vi "Pulse Generator 3.vi"(0 "Total Time":dbl=1500.0, 1 "EPR file path":path=path "C:/Users/Ouyang Group/Documents/Data/8-10-15/test", 3 "Z Pos":dbl=51.3, 4 "Pule Sequence file path":path=path "C:/Users/Ouyang Group/Documents/Data/8-6-15/T1 pulse sequence", 5 "X Pos":dbl=98.0, 7 "Y pos":dbl=76.0, 8 "start/restart":bool, 9 "track and epr":bool, 11 "Z-track?":bool, 12 "load":bool, 13 "Y Parameters":T1={"Number of Y Steps"=200, "Max Y (V)"=2.0, "Min Y (V)"=-2.0}, 16 "Tracking Interval":dbl=150.0, 17 "Tab Control":T3(tab)=enum."T1", 19 "X Parameters":T2={"Number of X Steps"=200, "Max X (V)"=2.0, "Min X (V)"=-2.0}, 20 "Rest time Min":dbl=2e-08, 21 "Rest time Max":dbl=0.0002, 25 "Rest time No. Steps":i32=20, 27 "type":u16(ring)=1 items=["Linear", "Logarithmic"]) -> (15 "Y Position":dbl=8.403706365395546, 23 "Z Position":dbl=77.35, 24 "X Position":dbl=39.29989668925261)   [LabVIEW 2012]
uses:
  <vilib>/Utility/file.llb/Write To Spreadsheet File (DBL).vi
panel:
  in  "CW for Tracking?":bool
  in  "Stop Program":bool
  out "EPR":bool
  out "Tracking Loop":dbl=6.0
  out "Track":bool
  out "Cross Section Y":dbl[](graph)=[21.0, 21.0, 22.0, 23.0, 28.0, 18.0, 27.0, 23.0, 21.0, 23.0, 27.0, 24.0, 27.0, 48.0, 72.0, 155.0, 223.0, 269.0, 346.0, 310.0, 298.0, 201.0, 115.0, 77.0, 45.0, 31.0, 30.0, 22.0, 20.0, 22.0, 23.0, 32.0, 17.0, 24.0, 22.0, 22.0, 31.0, 30.0, 37.0]
  out "Cross Section X":dbl[](graph)=[40.0, 23.0, 29.0, 30.0, 20.0, 26.0, 17.0, 31.0, 49.0, 64.0, 98.0, 144.0, 182.0, 231.0, 269.0, 259.0, 260.0, 248.0, 193.0, 187.0, 133.0, 113.0, 84.0, 52.0, 39.0, 24.0, 24.0, 33.0, 19.0, 20.0, 16.0, 21.0, 26.0, 30.0, 25.0, 26.0, 20.0, 24.0, 24.0]
  out "Gave up?":bool
  in  "RS232 settings":cluster{"Portnumber":i32, "Baudrate":u16}={"Portnumber"=6, "Baudrate"=5} {"Portnumber" items=["COM1", "COM2", "COM3", "COM4", "COM5", "COM6", "COM7", "COM8", "COM9", "COM10", "COM11", "COM12", "COM13", "COM14", "COM15", "COM16", "COM17", "COM18", "COM19", "COM20", "COM21", "COM22", "COM23", "COM24", "COM25", "COM26", "COM27", "COM28", "COM29", "COM30"]; "Baudrate" items=["9600", "14400", "19200", "38400", "57600", "115200"]}
  in  "ref?":bool=TRUE
  in  "MW Delay":dbl=5e-08
  in  "Sig/Ref pause":dbl=5e-07
  in  "Rate (Hz)":dbl=2.0
  in  "Pulse MW":bool
  in  "Pulse Laser":bool
  in  "Delay Blocks":u16=4
  in  "Divide By":u16(ring) items=["1", "8", "16", "32"]
  in  "MW width Min":dbl=2e-08
  in  "MW width step size":dbl=5e-09
  in  "MW width Max":dbl=5e-07
  in  "Rabi Freq":dbl=7000000.0
  in  "Tau Max":dbl=0.001
  in  "Tau Min":dbl=2e-08
  in  "Tau No. Steps":i32=20
  in  "type 2":u16(ring)=1 items=["Linear", "Logarithmic"]
  in  "T1 APD width":dbl=5e-07
  in  "T1 Signal Delay":dbl=6e-07
  in  "T1 AOM length":dbl=2.5e-06
  in  "T1 AOM Rest":dbl=1e-06
  in  "Pi Pulse?":bool
  in  "Tau step size":dbl
  in  "Tau max":dbl
  in  "Tau min":dbl
  in  "Rabi Frequency":dbl
  in  "Pulse offset 2":dbl
  in  "Rabi Frequency":dbl
  in  "Tau max":dbl
  in  "Tau min":dbl
  in  "Tau step size":dbl
  in  "Equal Pulse length":bool
  in  "Pulse offset":dbl
  in  "Tau":dbl
  in  "Rabi Frequency  2":dbl
  in  "Tau' max 2":dbl
  in  "Tau' min 2":dbl
  in  "Tau' step size 2":dbl
  in  "Rabi Frequency":dbl
  in  "Tau min":dbl
  in  "Tau max":dbl
  in  "Tau step size":dbl
  in  "No. Pi Pulses":i32
  in  "Pulse offset":dbl
  in  "0->+?":bool
  in  "AOM Rest time":dbl=1e-06
  in  "Signal delay":dbl=7.2e-07
  in  "N Loop":i32=10000
  in  "APD signal width":dbl=3e-07
  out "Run":bool
  out "Scan size":i32
  in  "AOM Pulse length":dbl=2.5e-06
  in  "Path to spinapi.dll":path=path "C:/SpinCore/SpinAPI/dll/spinapi64.dll"
  in  "stop":bool
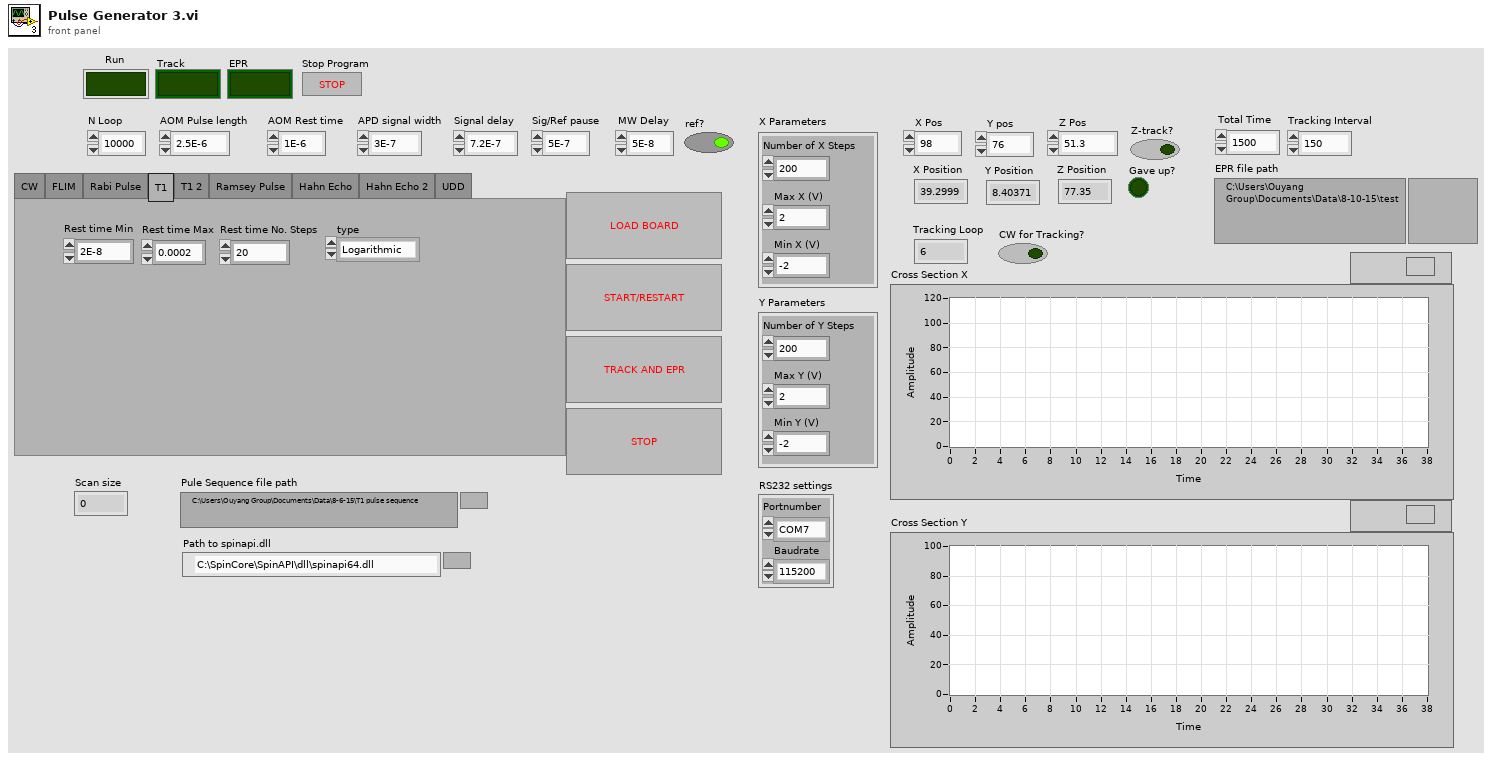
[diagram p1: front panel]
types:
  T1 = cluster{"Number of Y Steps":i32, "Max Y (V)":dbl, "Min Y (V)":dbl}
  T2 = cluster{"Number of X Steps":i32, "Max X (V)":dbl, "Min X (V)":dbl}
  T3 = enum32{"CW", "FLIM", "Rabi Pulse", "T1", "T1 2", "Ramsey Pulse", "Hahn Echo", "Hahn Echo 2", "UDD"}
  T4 = cluster{"Instruct Data":i32, "Op Code":i32, "Flags":bool[], "Comments":string, "Time (s)":dbl}
  T5 = enum16{"Pulse Program", "Frequency Registers", "TX Phase Registers", "RX Phase Registers"}
  T6 = cluster{"Instruct Data":i32, "Op Code":i32, "Flags":bool[], "Comments":string, "Time (s)":dbl}[]
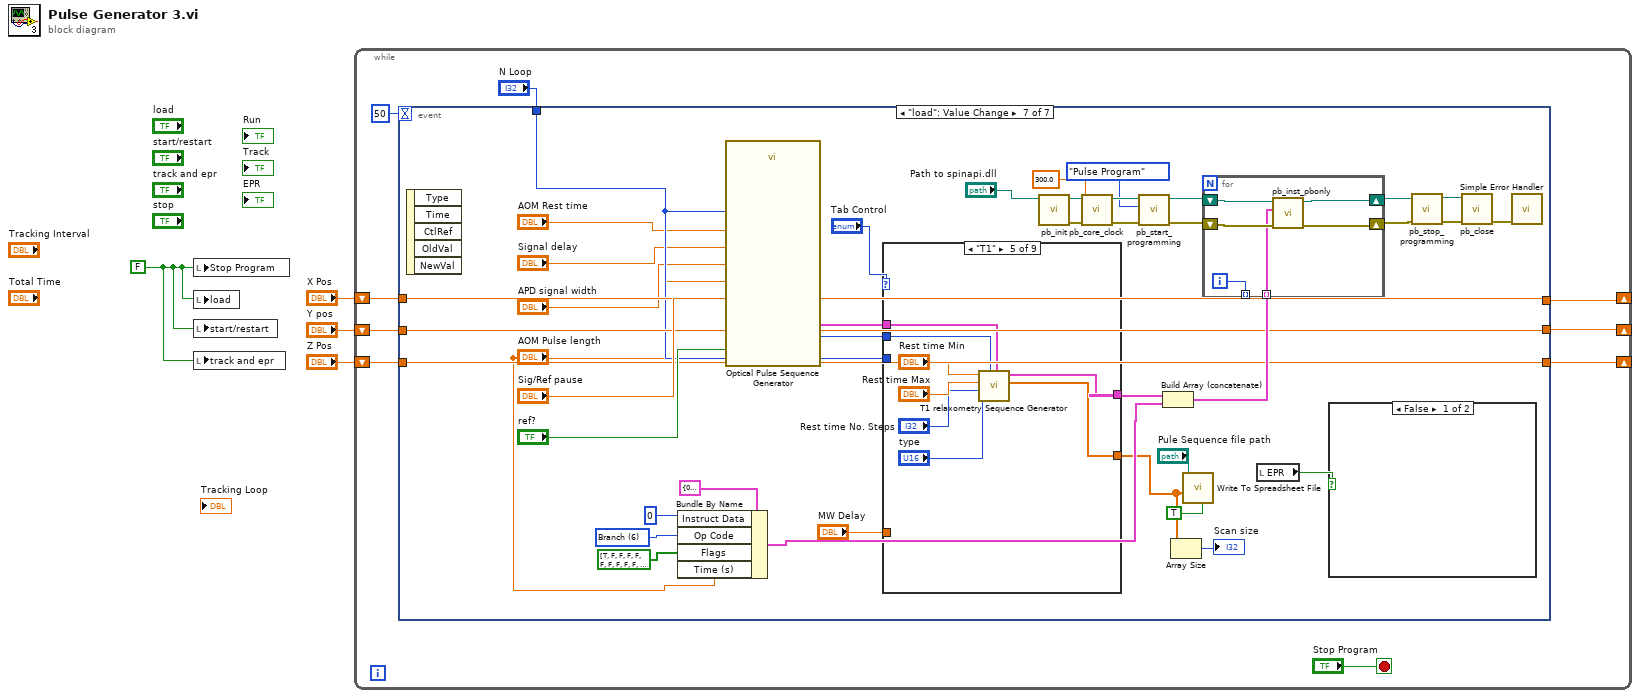
[diagram p0: block diagram]
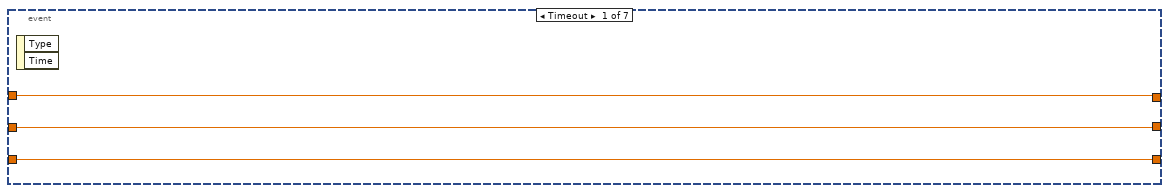
[diagram p2: hidden frame]
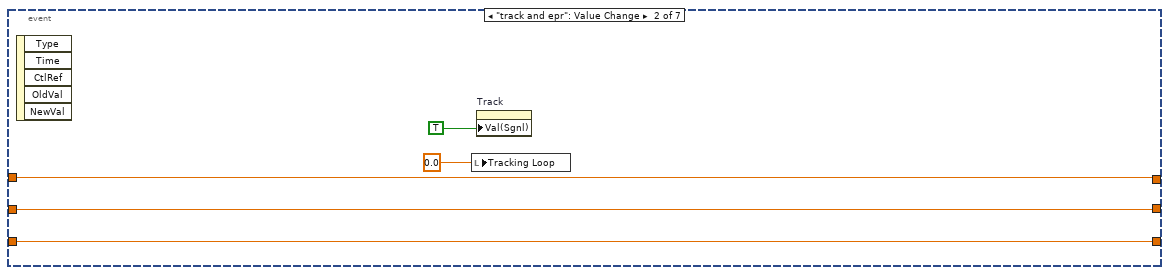
[diagram p3: hidden frame]
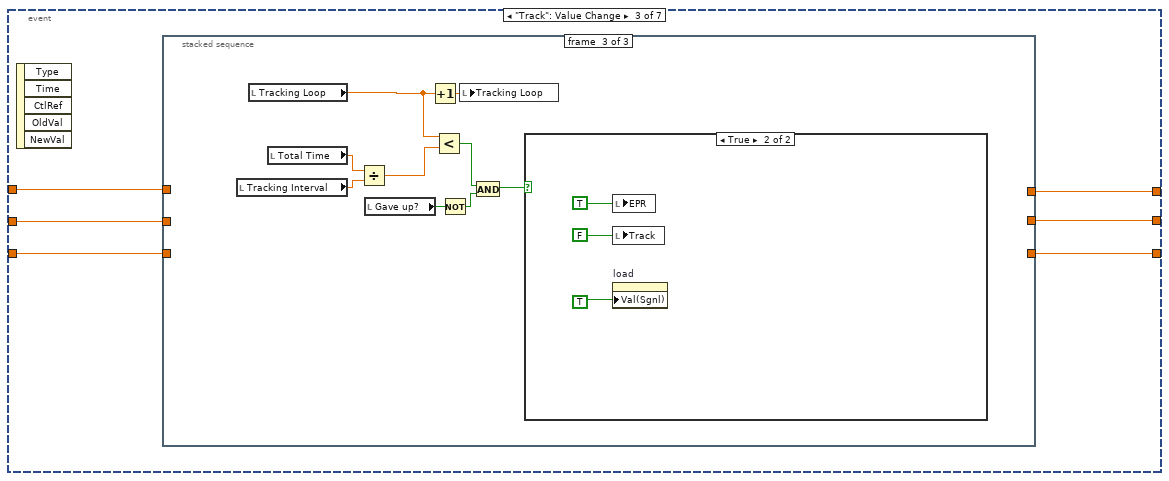
[diagram p4: hidden frame]
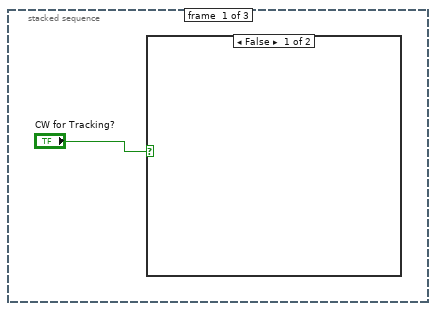
[diagram p5: hidden frame]
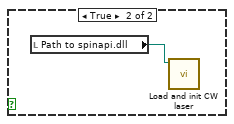
[diagram p6: hidden frame]
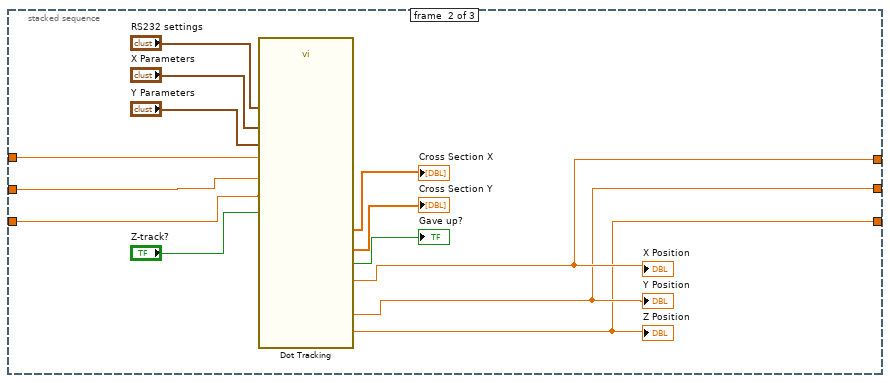
[diagram p7: hidden frame]
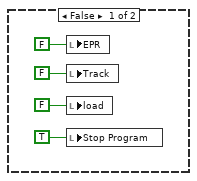
[diagram p8: hidden frame]
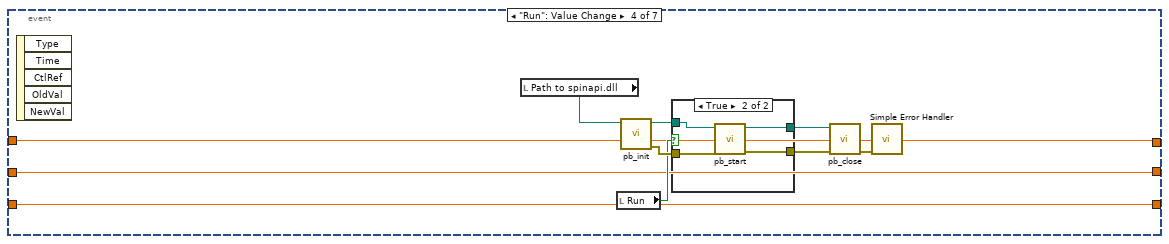
[diagram p9: hidden frame]
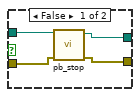
[diagram p10: hidden frame]
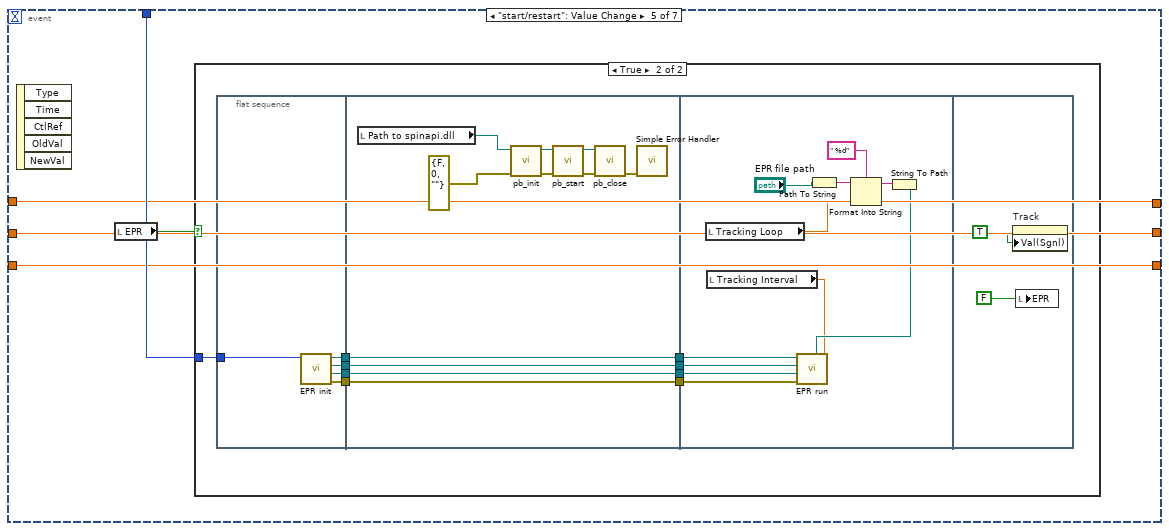
[diagram p11: hidden frame]
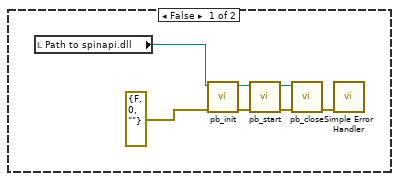
[diagram p12: hidden frame]
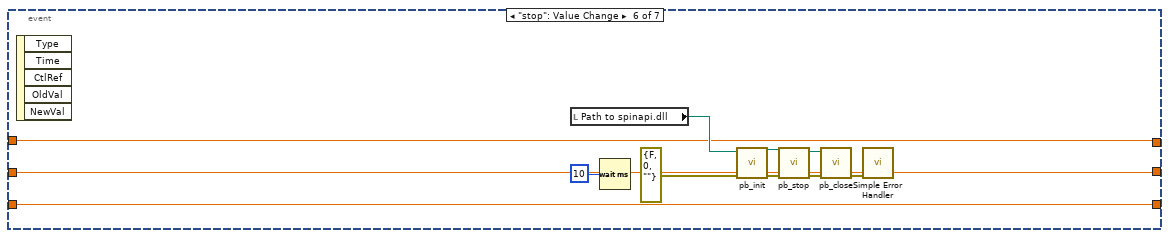
[diagram p13: hidden frame]
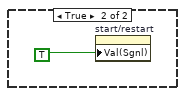
[diagram p14: hidden frame]
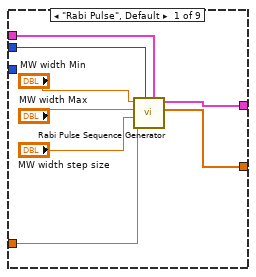
[diagram p15: hidden frame]
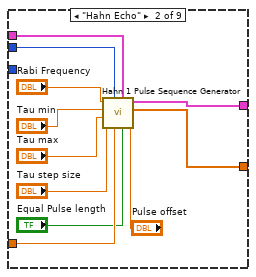
[diagram p16: hidden frame]
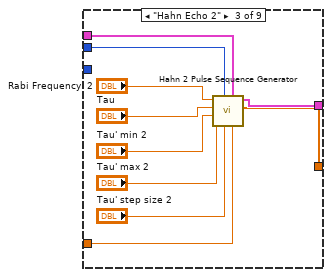
[diagram p17: hidden frame]
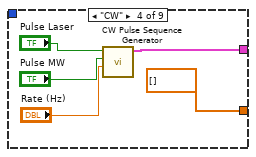
[diagram p18: hidden frame]
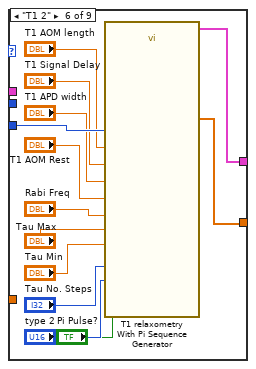
[diagram p19: hidden frame]
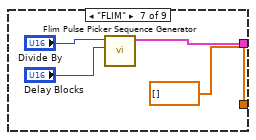
[diagram p20: hidden frame]
diagram:
  w4 = FALSE ("Stop Program")
  n1 = local write "Stop Program"(w4) -> ()
  n2 = local write "load"(w4) -> ()
  n3 = local write "start/restart"(w4) -> ()
  n4 = local write "track and epr"(w4) -> ()
  n5 = while {
    shift-right: [w7] -> _
    shift-left: "X Pos" -> [w10]
    shift-right: [w6] -> _
    shift-left: "Y pos" -> [w9]
    shift-right: [w5] -> _
    shift-left: "Z Pos" -> [w8]
    stop <- "Stop Program" stop-if-true
    n6 = event shown="[6] \"load\": Value Change" {
      selector: _ -> [_ _ _ _ _ _ _]
      dyn-events: _ -> [_ _ _ _ _ _ _]
      timeout: 50 -> [_ _ _ _ _ _ _]
      tunnel: "N Loop" -> [_ _ _ _ w80 _ w142]
      tunnel: w10 -> [w16 w19 w27 w61 w79 w129 w145]
      tunnel: w9 -> [w15 w18 w26 w60 w78 w128 w144]
      tunnel: w8 -> [w14 w17 w25 w59 w77 w127 w143]
      tunnel: [w16 w19 w24 w61 w79 w129 w145] -> w7
      tunnel: [w15 w18 w23 w60 w78 w128 w144] -> w6
      tunnel: [w14 w17 w22 w59 w77 w127 w143] -> w5
      event Timeout {
        n7 = event-data() -> ()  [unwired: 1 in, 2 out]
      }
      event "track and epr": Value Change {
        n8 = event-data() -> ()  [unwired: 1 in, 5 out]
        n9 = local write "Tracking Loop"(0.0 ("Tracking Loop")) -> ()
        n10 = property on="Track" class="Bool (strict)"("Val(Sgnl)"=TRUE ("Track")) -> ()  [unwired: 2 in, 2 out]
      }
      event "Track": Value Change {
        n11 = event-data() -> ()  [unwired: 1 in, 5 out]
        n12 = stacked-sequence {
          tunnel: w27 -> [_ w35 _]
          tunnel: w26 -> [_ w34 _]
          tunnel: w25 -> [_ w33 _]
          tunnel: [_ w32 _] -> w24
          tunnel: [_ w31 _] -> w23
          tunnel: [_ w30 _] -> w22
          frame #0 {
            n13 = case shown="False" "CW for Tracking?" {
              frame False {
              }
              frame True {
                n14 = local read "Path to spinapi.dll"() -> (w29:path)
                n15 = call "Load and init CW laser.vi"("path in"=w29) -> ()  [unwired: 11 in]
              }
            }
          }
          frame #1 {
            n16 = call "Dot Tracking.vi"("X"="X Parameters", "Y Parameters"="Y Parameters", "RS232 settings"="RS232 settings", "X Pos"=w35, "Y pos"=w34, "Z Pos"=w33, "Z-track?"="Z-track?") -> ("X Position"=w32:dbl, "Y Position"=w31:dbl, "Z Position"=w30:dbl, "Cross Section X"=→"Cross Section X":dbl[], "Cross Section Y"=→"Cross Section Y":dbl[], "Gave up?"=→"Gave up?":bool)  [unwired: 2 in, 1 out]
            "X Position" <- w32
            "Y Position" <- w31
            "Z Position" <- w30
          }
          frame #2 {
            n17 = local read "Tracking Interval"() -> (w51:dbl)
            n18 = local read "Tracking Loop"() -> (w44:dbl)
            n19 = local read "Total Time"() -> (w50:dbl)
            n20 = Divide(x=w50, y=w51) -> (x/y=w49:dbl)
            n21 = local read "Gave up?"() -> (w47:bool)
            n22 = Increment(x=w44) -> (x+1=w43:dbl)
            n23 = Less?(x=w44, y=w49) -> (x < y?=w48:bool)
            n24 = Not(x=w47) -> (.not. x?=w45:bool)
            n25 = local write "Tracking Loop"(w43) -> ()
            n26 = And(x=w48, y=w45) -> (x .and. y?=w46:bool)
            n27 = case shown="True" w46 {
              frame False {
                n28 = local write "EPR"(FALSE ("EPR")) -> ()
                n29 = local write "Track"(FALSE ("Track")) -> ()
                n30 = local write "load"(FALSE ("load")) -> ()
                n31 = local write "Stop Program"(TRUE ("Stop Program")) -> ()
              }
              frame True {
                n32 = local write "EPR"(TRUE ("EPR")) -> ()
                n33 = local write "Track"(FALSE ("Track")) -> ()
                n34 = property on="load" class="Bool (strict)"("Val(Sgnl)"=TRUE ("load")) -> ()  [unwired: 2 in, 2 out]
              }
            }
          }
        }
      }
      event "Run": Value Change {
        n35 = event-data() -> ()  [unwired: 1 in, 5 out]
        n36 = local read "Path to spinapi.dll"() -> (w62:path)
        n37 = local read "Run"() -> (w66:bool)
        n38 = call "pb_init.vi"("path in"=w62) -> ("error out"=w67:errorcluster, "path out"=w68:path)  [unwired: 2 in, 7 out]
        n39 = case shown="True" w66 {
          tunnel: w68 -> [w72 w76]
          tunnel: w67 -> [w71 w75]
          tunnel: [w70 w74] -> w64
          tunnel: [w69 w73] -> w63
          frame False {
            n40 = call "pb_stop.vi"("error in (no error)"=w71, "path in"=w72) -> ("error out"=w69:errorcluster, "path out"=w70:path)  [unwired: 8 out]
          }
          frame True {
            n41 = call "pb_start.vi"("error in (no error)"=w75, "path in"=w76) -> ("error out"=w73:errorcluster, "path out"=w74:path)  [unwired: 1 in, 7 out]
          }
        }
        n42 = call "pb_close.vi"("error in (no error)"=w63, "path in"=w64) -> ("error out"=w65:errorcluster)  [unwired: 9 out]
        n43 = call <vilib>:"Simple Error Handler.vi"("error in (no error)"=w65) -> ()  [unwired: 1 in, 8 out]
      }
      event "start/restart": Value Change {
        n44 = event-data() -> ()  [unwired: 1 in, 5 out]
        n45 = local read "EPR"() -> (w81:bool)
        n46 = case shown="True" w81 {
          tunnel: w80 -> [_ w89]
          frame False {
            n47 = local read "Path to spinapi.dll"() -> (w83:path)
            n48 = call "pb_init.vi"("error in (no error)"=errorcluster {"status"=FALSE, "code"=0, "source"=""}, "path in"=w83) -> ("error out"=w86:errorcluster, "path out"=w84:path)  [unwired: 1 in, 7 out]
            n49 = call "pb_start.vi"("error in (no error)"=w86, "path in"=w84) -> ("error out"=w87:errorcluster, "path out"=w82:path)  [unwired: 1 in, 7 out]
            n50 = call "pb_close.vi"("error in (no error)"=w87, "path in"=w82) -> ("error out"=w88:errorcluster)  [unwired: 9 out]
            n51 = call <vilib>:"Simple Error Handler.vi"("error in (no error)"=w88) -> ()  [unwired: 1 in, 8 out]
          }
          frame True {
            n52 = flat-sequence {
              tunnel: [w102] -> w96
              tunnel: [w101] -> w94
              tunnel: [w100] -> w92
              tunnel: [w99] -> w90
              tunnel: w89 -> [w98]
              tunnel: [w106] -> w97
              tunnel: w96 -> [w106]
              tunnel: [w105] -> w95
              tunnel: w94 -> [w105]
              tunnel: [w104] -> w93
              tunnel: w92 -> [w104]
              tunnel: [w103] -> w91
              tunnel: w90 -> [w103]
              tunnel: w97 -> [w117]
              tunnel: w95 -> [w116]
              tunnel: w93 -> [w115]
              tunnel: w91 -> [w114]
              frame #0 {
                n53 = call "EPR init.vi"("N loops"=w98) -> ("error out"=w99:errorcluster, "ref task out"=w100:refnum<k21>, "sig task out"=w101:refnum<k21>, "clock task out"=w102:refnum<k21>)  [unwired: 7 in]
              }
              frame #1 {
                n54 = local read "Path to spinapi.dll"() -> (w113:path)
                n55 = call "pb_init.vi"("error in (no error)"=errorcluster {"status"=FALSE, "code"=0, "source"=""}, "path in"=w113) -> ("error out"=w110:errorcluster, "path out"=w108:path)  [unwired: 1 in, 7 out]
                n56 = call "pb_start.vi"("error in (no error)"=w110, "path in"=w108) -> ("error out"=w111:errorcluster, "path out"=w107:path)  [unwired: 1 in, 7 out]
                n57 = call "pb_close.vi"("error in (no error)"=w111, "path in"=w107) -> ("error out"=w112:errorcluster)  [unwired: 9 out]
                n58 = call <vilib>:"Simple Error Handler.vi"("error in (no error)"=w112) -> ()  [unwired: 1 in, 8 out]
              }
              frame #2 {
                n59 = local read "Tracking Loop"() -> (w120:dbl)
                n60 = local read "Tracking Interval"() -> (w118:dbl)
                n61 = Path To String(path="EPR file path") -> (string=w123:string)
                n62 = Format Into String(format string=" %d", initial string=w123, w120) -> (resulting string=w122:string)  [unwired: 1 in, 1 out]
                n63 = String To Path(string=w122) -> (path=w119:path)
                n64 = call "EPR run.vi"("control task in"=w117, "sig task in"=w116, "ref task in"=w115, "error in"=w114, "file path (dialog if empty)"=w119, "Measurement Interval"=w118) -> ()  [unwired: 4 in]
              }
              frame #3 {
                n65 = property on="Track" class="Bool (strict)"("Val(Sgnl)"=TRUE ("Track")) -> ()  [unwired: 2 in, 2 out]
                n66 = local write "EPR"(FALSE ("EPR")) -> ()
              }
            }
          }
        }
      }
      event "stop": Value Change {
        n67 = event-data() -> ()  [unwired: 1 in, 5 out]
        n68 = local read "Path to spinapi.dll"() -> (w136:path)
        n69 = Wait (ms)(milliseconds to wait=u32 10) -> ()  [unwired: 1 out]
        n70 = call "pb_init.vi"("error in (no error)"=errorcluster {"status"=FALSE, "code"=0, "source"=""}, "path in"=w136) -> ("error out"=w133:errorcluster, "path out"=w131:path)  [unwired: 1 in, 7 out]
        n71 = call "pb_stop.vi"("error in (no error)"=w133, "path in"=w131) -> ("error out"=w134:errorcluster, "path out"=w130:path)  [unwired: 8 out]
        n72 = call "pb_close.vi"("error in (no error)"=w134, "path in"=w130) -> ("error out"=w135:errorcluster)  [unwired: 9 out]
        n73 = call <vilib>:"Simple Error Handler.vi"("error in (no error)"=w135) -> ()  [unwired: 1 in, 8 out]
      }
      event "load": Value Change {
        w169 = 6 items=["Continue", "Stop", "Loop", "End Loop", "JSR", "RTS", "Branch", "Long Delay", "Wait"] ("Op Code")
        n74 = event-data() -> ()  [unwired: 1 in, 5 out]
        n75 = Bundle By Name(cluster=T4 {"Instruct Data"=0, "Op Code"=0, "Flags"=[FALSE, FALSE, FALSE, FALSE, FALSE, FALSE, FALSE, FALSE, FALSE, FALSE, FALSE, FALSE, FALSE, FALSE, FALSE, FALSE, FALSE, FALSE, FALSE, FALSE, FALSE, TRUE, TRUE, TRUE], "Comments"="", "Time (s)"=0.01} ("PB Inst 2"), "Instruct Data"=0, "Op Code"=w169, "Flags"=bool[] [TRUE, FALSE, FALSE, FALSE, FALSE, FALSE, FALSE, FALSE, FALSE, FALSE, FALSE, FALSE, FALSE, FALSE, FALSE, FALSE, FALSE, FALSE, FALSE, FALSE, FALSE, TRUE, TRUE, TRUE], "Time (s)"="AOM Pulse length") -> (w177:T4)
        n76 = call "Optical Pulse Sequence Generator.vi"("ref?"="ref?", "N Loop"=w142, "Sig/Ref pause"="Sig/Ref pause", "AOM Rest time"="AOM Rest time", "Signal delay"="Signal delay", "APD signal width"="APD signal width", "AOM Pulse length"="AOM Pulse length") -> ("Array"=w172:T6, "No. Instructions"=w173:i32)  [unwired: 3 in]
        n77 = case shown="\"T1\"" "Tab Control" {
          tunnel: w172 -> [w181 w191 w200 _ w219 _ _ w248 w257]
          tunnel: w173 -> [w182 w192 w201 _ w220 _ _ w249 w256]
          tunnel: "MW Delay" -> [w183 w193 w202 _ _ _ _ w241 w251]
          tunnel: [w180 w190 w199 w209 w218 w227 w237 w247 w258] -> w176
          tunnel: [w179 w189 w198 dbl[] [] ("Tau") w217 w226 dbl[] [] ("Tau") w246 w259] -> w167
          tunnel: w142 -> [_ _ _ _ _ w233 _ _ _]
          frame "Rabi Pulse", Default {
            n78 = call "Rabi Pulse Sequence Generator.vi"("Optical Pulse"=w181, "No. Instructions"=w182, "MW Delay"=w183, "MW width step size"="MW width step size", "MW width Max"="MW width Max", "MW width Min"="MW width Min") -> ("Pulse Width"=w179:dbl[], "Pulse Sequence Out"=w180:T6)  [unwired: 4 in]
          }
          frame "Hahn Echo" {
            n79 = call "Hahn 1 Pulse Sequence Generator.vi"("Pulse offset"="Pulse offset", "Equal Pulse length"="Equal Pulse length", "Array"=w191, "MW Delay"=w193, "No. Instructions"=w192, "Tau step size"="Tau step size", "Tau max"="Tau max", "Tau min"="Tau min", "Rabi Frequency"="Rabi Frequency") -> ("Tau"=w189:dbl[], "Pulse Sequence"=w190:T6)  [unwired: 1 in]
          }
          frame "Hahn Echo 2" {
            n80 = call "Hahn 2 Pulse Sequence Generator.vi"("MW Delay"=w202, "Optical Pulse Sequence"=w200, "Tau' step size 2"="Tau' step size 2", "No. Instructions"=w201, "Tau' max 2"="Tau' max 2", "Tau' min 2"="Tau' min 2", "Tau"="Tau", "Rabi Frequency  2"="Rabi Frequency  2") -> ("Tau'"=w198:dbl[], "Pulse Sequence"=w199:T6)  [unwired: 2 in]
          }
          frame "CW" {
            n81 = call "CW Pulse Sequence Generator.vi"("Pulse Laser"="Pulse Laser", "Pulse MW"="Pulse MW", "Rate (Hz)"="Rate (Hz)") -> ("Pulse Sequence Out"=w209:T6)  [unwired: 7 in]
          }
          frame "T1" {
            n82 = call "T1 relaxometry Sequence Generator.vi"("Optical Pulse"=w219, "No. Instructions"=w220, "type"="type", "Rest time No. Steps"="Rest time No. Steps", "Rest time Max"="Rest time Max", "Rest time Min"="Rest time Min") -> ("Pulse Width"=w217:dbl[], "Pulse Sequence Out"=w218:T6)  [unwired: 4 in]
          }
          frame "T1 2" {
            n83 = call "T1 relaxometry With Pi Sequence Generator.vi"("N Loop"=w233, "AOM Pulse length"="T1 AOM length", "AOM Rest time"="T1 AOM Rest", "Signal Delay"="T1 Signal Delay", "APD signal width"="T1 APD width", "Rabi Freq"="Rabi Freq", "Pi Pulse?"="Pi Pulse?", "Tau Min"="Tau Min", "Tau Max"="Tau Max", "Tau No. Steps"="Tau No. Steps", "type"="type 2") -> ("Array"=w227:T6, "Tau Pattern"=w226:dbl[])  [unwired: 7 in]
          }
          frame "FLIM" {
            n84 = call "Flim Pulse Picker Sequence Generator.vi"("Delay Blocks"="Delay Blocks", "Divide By"="Divide By") -> ("Pulse Sequence Out"=w237:T6)  [unwired: 9 in]
          }
          frame "UDD" {
            n85 = call "UDD Pulse Sequence Generator.vi"("Rabi Frequency"="Rabi Frequency", "No. Instructions"=w249, "Array"=w248, "Tau min"="Tau min", "Tau max"="Tau max", "Tau step size"="Tau step size", "MW Delay"=w241, "0->+?"="0->+?", "No. Pi Pulses"="No. Pi Pulses", "Pulse offset"="Pulse offset") -> ("Pulse Sequence"=w247:T6, "Tau"=w246:dbl[])  [unwired: 4 in]
          }
          frame "Ramsey Pulse" {
            n86 = call "Ramsey Pulse Sequence Generator.vi"("Pulse offset"="Pulse offset 2", "Array"=w257, "MW Delay"=w251, "No. Instructions"=w256, "Tau step size"="Tau step size", "Tau max"="Tau max", "Tau min"="Tau min", "Rabi Frequency"="Rabi Frequency") -> ("Tau"=w259:dbl[], "Pulse Sequence"=w258:T6)  [unwired: 2 in]
          }
        }
        n87 = call "pb_init.vi"("path in"="Path to spinapi.dll") -> ("error out"=w154:errorcluster, "path out"=w152:path)  [unwired: 3 in, 6 out]
        n88 = call "pb_core_clock.vi"("error in (no error)"=w154, "clock_freq (MHz)"=300.0, "path in"=w152) -> ("error out"=w155:errorcluster, "path out"=w153:path)  [unwired: 7 in]
        n89 = call "pb_start_programming.vi"("error in (no error)"=w155, "Device"=T5."Pulse Program", "path in"=w153) -> ("error out"=w158:errorcluster, "path out"=w157:path)  [unwired: 1 in, 6 out]
        n90 = Build Array (concatenate)(w176, w177) -> (w166:T6)
        n91 = Array Size(array=w167) -> (size(s)=→"Scan size":i32)
        n92 = call-poly <vilib>:"Write To Spreadsheet File.vi"("transpose? (no:F)"=TRUE, "1D data"=w167, "file path (dialog if empty)"="Pule Sequence file path") -> ()  [unwired: 5 in, 1 out]
        n93 = for {
          shift-right: [w263] -> w159
          shift-left: w157 -> [w265]
          shift-right: [w262] -> w160
          shift-left: w158 -> [w264]
          tunnel: [w261] -> _ mode=indexing
          tunnel: w166 -> [w260] mode=indexing
          i -> [w261]
          n94 = call "pb_inst_pbonly.vi"("error in (no error)"=w264, "PB Instruction"=w260, "path in"=w265) -> ("error out"=w262:errorcluster, "path out"=w263:path)  [unwired: 2 in, 5 out]
        }
        n95 = local read "EPR"() -> (w146:bool)
        n96 = case shown="False" w146 {
          frame False {
          }
          frame True {
            n97 = property on="start/restart" class="Bool (strict)"("Val(Sgnl)"=TRUE ("start/restart")) -> ()  [unwired: 2 in, 2 out]
          }
        }
        n98 = call "pb_stop_programming.vi"("error in (no error)"=w160, "path in"=w159) -> ("error out"=w151:errorcluster, "path out"=w150:path)  [unwired: 1 in, 7 out]
        n99 = call "pb_close.vi"("error in (no error)"=w151, "path in"=w150) -> ("error out"=w162:errorcluster)  [unwired: 9 out]
        n100 = call <vilib>:"Simple Error Handler.vi"("error in (no error)"=w162) -> ()  [unwired: 1 in, 8 out]
      }
    }
  }
